vi "controlRealTimeInChangePerPulse.vi"(7 "Set":bool, 8 "error in":errorcluster, 9 "Change in":i32, 10 "axis in":u8, 11 "connection ID":i32) -> (0 "error out":errorcluster, 1 "Change out":i32, 2 "axis out":u8, 3 "connection ID":i32)   [LabVIEW 2016]
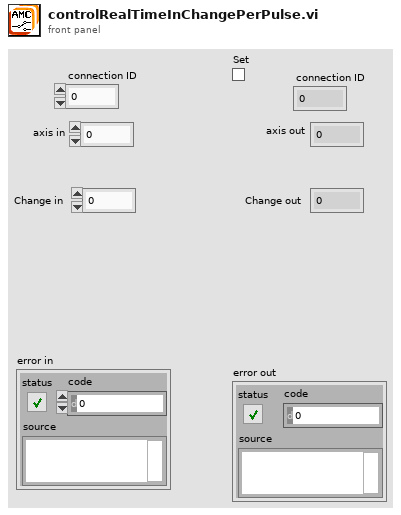
[diagram p1: front panel]
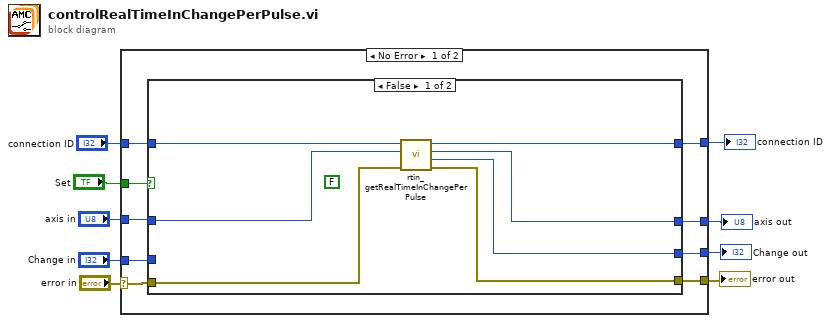
[diagram p0: block diagram]
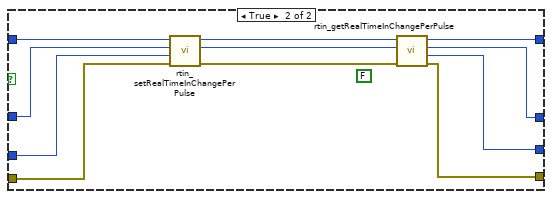
[diagram p2: hidden frame]
diagram:
  n1 = case shown="No Error" "error in" {
    selector: "error in" -> [w10 w40]
    tunnel: "axis in" -> [w17 w38]
    tunnel: [w11 w40] -> w8
    tunnel: [w13 w38] -> w7
    tunnel: "Set" -> [w18 _]
    tunnel: [w14 w37] -> w5
    tunnel: "connection ID" -> [w15 w37]
    tunnel: "Change in" -> [w16 w39]
    tunnel: [w12 w39] -> w2
    frame No Error {
      n2 = case shown="False" w18 {
        tunnel: [w24 w28] -> w14
        tunnel: w15 -> [w25 w36]
        tunnel: w17 -> [w20 w33]
        tunnel: [w23 w27] -> w13
        tunnel: [w22 w31] -> w11
        tunnel: [w19 w26] -> w12
        tunnel: w16 -> [_ w34]
        tunnel: w10 -> [w21 w35]
        frame False {
          (unwired) FALSE ("tempvalue")
          n3 = call "rtin_getRealTimeInChangePerPulse.vi"("error in"=w21, "axis"=w20, "connection ID"=w25) -> ("error out"=w22:errorcluster, "resolution"=w19:i32, "axis_out"=w23:i32, "connection ID"=w24:i32)  [unwired: 5 in]
        }
        frame True {
          (unwired) FALSE ("tempvalue")
          n4 = call "rtin_setRealTimeInChangePerPulse.vi"("error in"=w35, "delta"=w34, "axis"=w33, "connection ID"=w36) -> ("error out"=w32:errorcluster, "axis_out"=w29:i32, "connection ID"=w30:i32)  [unwired: 5 in]
          n5 = call "rtin_getRealTimeInChangePerPulse.vi"("error in"=w32, "axis"=w29, "connection ID"=w30) -> ("error out"=w31:errorcluster, "resolution"=w26:i32, "axis_out"=w27:i32, "connection ID"=w28:i32)  [unwired: 5 in]
        }
      }
    }
    frame Error {
    }
  }
  "error out" <- w8
  "axis out" <- w7
  "connection ID" <- w5
  "Change out" <- w2
